vi "mul priority.vi"() -> ()   [LabVIEW 2020]
uses:
  <vilib>/Analysis/Matrix/Datatypes/RealMatrix.ctl
  <vilib>/Platform/TimedLoop/XDataNode/timing_clust.ctl
  <vilib>/Platform/TimedLoop/XDataNode/nitl_modes.ctl
  <vilib>/Platform/TimedLoop/XDataNode/wakeup.ctl
  <vilib>/Analysis/Matrix/Numeric/Conversions/Array To Matrix - RA.vi
  <vilib>/Analysis/Matrix/Numeric/Conversions/Array To Matrix - RA2.vi
  <vilib>/Analysis/Matrix/Numeric/Multiply/Multiply - RM,RM.vi
  <vilib>/platform/TimedLoop/XDataNode/XDataNode.xnode
  <vilib>/Analysis/Matrix/NI_Matrix.lvlib
  <vilib>/Platform/TimedLoop/XDataNode/XDNodeRunTimeDep.lvlib
panel:
  out "overall time":u32
  out "product":T1
  in  "vector size":i32=20
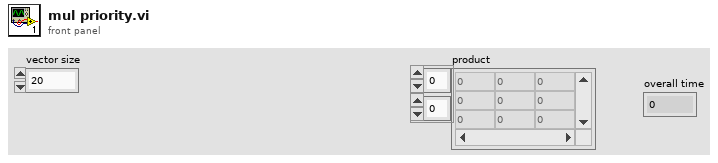
[diagram p1: front panel]
types:
  T1 = typedef "NI_Matrix.lvlib/RealMatrix.ctl" = dbl[][]
  T2 = typedef "XDNodeRunTimeDep.lvlib/timing_clust.ctl" = cluster{"Expected End [f-1]":u64, "Actual End [f-1]":u64, "Finished Late? [f-1]":bool, "Expected End [i-1]":u64, "Actual End [i-1]":u64, "Finished Late? [i-1]":bool, "Expected Start [i]":u64, "Actual Start [i]":u64, "Expected Start [f]":u64, "Actual Start [f]":u64, "Source Name":string, "Structure Name":string, "Period":i64, "Deadline":i64, "Offset":i64, "Start":i64, "Priority":i32, "Timeout":i32, "Mode":T3, "Wakeup Reason":T4, "Error":errorcluster, "Source Type":string, "Secondary Source Type":string, "Global End Time":u64, "Global Start Time":u64, "Frame Duration":u64, "Iteration Duration":u64, "Assigned CPU":i32, "I/O Scan Engine Mode":u32}
  T3 = typedef "XDNodeRunTimeDep.lvlib/nitl_modes.ctl" = enum32{"No Change", "Process missed periods, maintain original phase", "Discard missed periods, maintain original phase", "Process missed periods, ignore original phase", "Discard missed periods, ignore original phase"}
  T4 = typedef "XDNodeRunTimeDep.lvlib/wakeup.ctl" = enum32{"Normal", "Aborted", "Asynchronous wakeup", "Timing source error", "Timed loop error", "Timeout"}
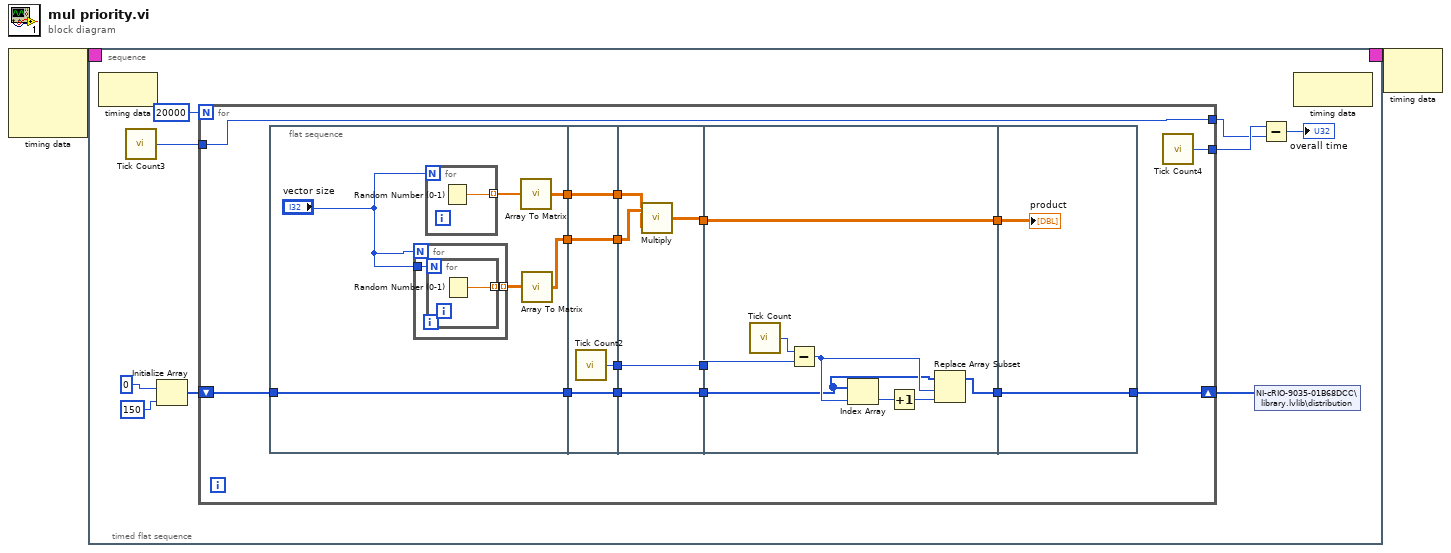
[diagram p0: block diagram]
diagram:
  n1 = node-c288() -> (w2:T2)  [unwired: 4 in]
  n2 = timed-sequence {
    timing: w2 -> [_]
    timing-out: [_] -> w1
    n3 = timed-flat-sequence {
      n4 = node-c288() -> ()  [unwired: 1 in, 1 out]
      n5 = call "Tick Count3"() -> ("Tick Count(uSec)"=w7:u32)
      n6 = Initialize Array(0, 150) -> (w8:i32[])
      n7 = for {
        N: 20000 -> [_]
        shift-right: [w14] -> w3
        shift-left: w8 -> [w16]
        tunnel: [w13] -> w5
        tunnel: w7 -> [w13]
        tunnel: [w12] -> w6
        n8 = flat-sequence {
          tunnel: [w32] -> w27
          tunnel: [w30] -> w21
          tunnel: [w28] -> w17
          tunnel: w16 -> [w28]
          tunnel: w27 -> [w41]
          tunnel: [w41] -> w26
          tunnel: [w40] -> w25
          tunnel: [w39] -> w22
          tunnel: w21 -> [w39]
          tunnel: [w38] -> w18
          tunnel: w17 -> [w38]
          tunnel: w26 -> [w44]
          tunnel: w25 -> [w46]
          tunnel: [w46] -> w24
          tunnel: [w43] -> w23
          tunnel: w22 -> [w45]
          tunnel: [w42] -> w19
          tunnel: w18 -> [w42]
          tunnel: w23 -> [w52]
          tunnel: w24 -> [w53]
          tunnel: [w52] -> w20
          tunnel: w19 -> [w48]
          tunnel: [w47] -> w15
          tunnel: w20 -> [w56]
          tunnel: w15 -> [w55]
          tunnel: [w55] -> w14
          frame #0 {
            n9 = for {
              N: "vector size" -> [_]
              tunnel: [w35] -> w31 mode=indexing
              tunnel: "vector size" -> [w34]
              n10 = for {
                N: w34 -> [_]
                tunnel: [w36] -> w35 mode=indexing
                n11 = Random Number (0-1)() -> (number: 0 to 1=w36:dbl)
              }
            }
            n12 = for {
              N: "vector size" -> [_]
              tunnel: [w37] -> w33 mode=indexing
              n13 = Random Number (0-1)() -> (number: 0 to 1=w37:dbl)
            }
            n14 = call-poly <vilib>:"Array To Matrix.vi"("Real 1D Array"=w33) -> ("Real Matrix (Column Vector)"=w32:T1)
            n15 = call-poly <vilib>:"Array To Matrix.vi"("Real 2D Array"=w31) -> ("Real Matrix"=w30:T1)
          }
          frame #1 {
            n16 = call "Tick Count2"() -> ("Tick Count(uSec)"=w40:u32)
          }
          frame #2 {
            n17 = call-poly <vilib>:"Multiply.vi"("Real Matrix B"=w44, "Real Matrix A"=w45) -> ("A * B"=w43:T1)
          }
          frame #3 {
            n18 = call "Tick Count"() -> ("Tick Count(uSec)"=w54:u32)
            n19 = Subtract(x=w54, y=w53) -> (x-y=w49:u32)
            n20 = Index Array(array=w48, index=w49) -> (element=w50:i32)
            n21 = Increment(x=w50) -> (x+1=w51:i32)
            n22 = Replace Array Subset(array=w48, new element=w51, index=w49) -> (w47:i32[])
          }
          frame #4 {
            "product" <- w56
          }
        }
        n23 = call "Tick Count4"() -> ("Tick Count(uSec)"=w12:u32)
      }
      n24 = shared-variable "NI-cRIO-9035-01B68DCC\\library.lvlib\\distribution"(w3) -> ()  [unwired: 1 in, 1 out]
      n25 = Subtract(x=w6, y=w5) -> (x-y=→"overall time":u32)
      n26 = node-c288() -> ()  [unwired: 1 in, 1 out]
    }
  }
  n27 = node-c288(w1) -> ()  [unwired: 1 out]
